vi "Solution Average 3.vi"(1 "Input 3":dbl, 2 "Input 2":dbl, 3 "Input 1":dbl) -> (0 "Output":dbl)   [LabVIEW 2019]
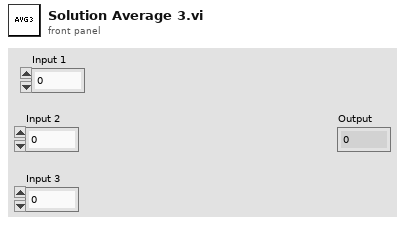
[diagram p1: front panel]
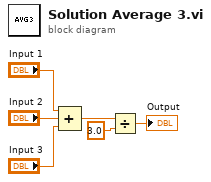
[diagram p0: block diagram]
diagram:
  n1 = Compound Arithmetic op=ADD("Input 1", "Input 2", "Input 3") -> (w3:dbl)
  n2 = Divide(x=w3, y=3.0) -> (x/y=→"Output":dbl)
